vi "7L13-c-CSM.vi"(5 "err in":errorcluster, 8 "Coût (e)":T2, 9 "Pièce (e)":T1) -> (2 "Coût (s)":T2, 4 "err out":errorcluster)   [LabVIEW 2010, in "lv_07.lvlib"]
doc: "Calcul des coûts de stockage Maintenance (CSM)"
uses:
  lv_07.lvlib
  c_cout_choix_q.ctl
  c_pi_wilson.ctl
panel:
  out "Pièce (s)":T1
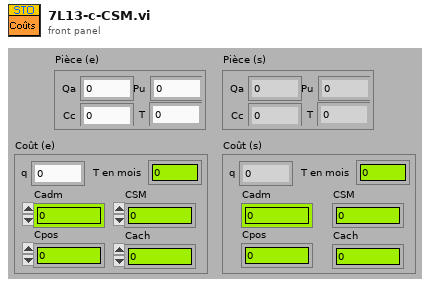
[diagram p1: front panel]
types:
  T1 = typedef "lv_07.lvlib/c_pi_wilson.ctl" = cluster{"T":dbl, "Pu":dbl, "Qa":dbl, "Cc":dbl}
  T2 = typedef "lv_07.lvlib/c_cout_choix_q.ctl" = cluster{"Cadm":dbl, "Cpos":dbl, "Cach":dbl, "CSM":dbl, "q":dbl, "T en mois":dbl}
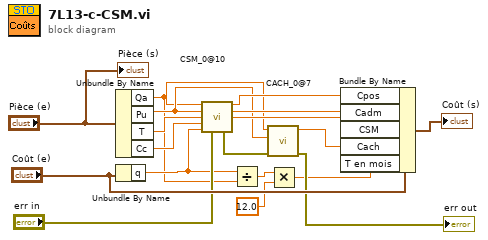
[diagram p0: block diagram]
diagram:
  n1 = Unbundle By Name("Pièce (e)") -> ("Qa"=w4:dbl, "Pu"=w7:dbl, "T"=w11:dbl, "Cc"=w10:dbl)
  n2 = Unbundle By Name("Coût (e)") -> ("q"=w5:dbl)
  n3 = call "CSM_0@10.vi"("Qa"=w4, "Pu"=w7, "T"=w11, "Cc"=w10, "q"=w5, "err in"="err in") -> ("Cpos"=w14:dbl, "Cadm"=w13:dbl, "CSM"=w15:dbl, "err out"=w9:errorcluster)  [unwired: 6 in]
  n4 = Divide(x=w5, y=w4) -> (x/y=w3:dbl)
  n5 = call "CACH_0@7.vi"("err in"=w9, "Pu"=w7, "Qa"=w4) -> ("err out"=→"err out":errorcluster, "Cach"=w17:dbl)  [unwired: 5 in]
  n6 = Multiply(x=w3, y=12.0) -> (x*y=w1:dbl)
  n7 = Bundle By Name(cluster="Coût (e)", "Cpos"=w14, "Cadm"=w13, "CSM"=w15, "Cach"=w17, "T en mois"=w1) -> (→"Coût (s)":T2)
  "Pièce (s)" <- "Pièce (e)"
